vi "LABVIEW.vi"() -> ()   [LabVIEW 2017]
uses:
  <vilib>/picture/picture.llb/imagedata.ctl
  <vilib>/Instr/_visa.llb/VISA Configure Serial Port (Instr).vi
  <vilib>/Utility/file.llb/Write To Spreadsheet File (DBL).vi
panel:
  out "image data 2":T1
  out "image data":T1
  in  "Tab Control":enum32{"CONFIGURAÇÃO", "ANÁLISE", "DEBUG"}(tab)
  in  "ARQUIVO DE DADOS":path
  in  "PORTA COM":refnum<visa-resource-name>
  in  "BAUD RATE (9600)":u32=9600
  in  "TEMPO (ms)":u32
  out "new picture 2":picture
  in  "IMAGEM DA ABA CONFIGURAÇÃO":path
  in  "IMAGEM DA ABA DEBUG":path
  in  "GRAVAR":bool
  out "TEMPO (s)":dbl
  out "GRÁFICO \nTEMPERATURA":dbl(graph)
  out "TEMPERATURA":dbl
  in  "?":bool
  in  "POTÊNCIA \nRESISTÊNCIA":dbl(slide) scale=0.0..100.0
  out "?":string
  out "?":string
  out "new picture":picture
  # "ARQUIVO EM QUE OS DADOS DEVERÃO SER GRAVADOS"
  # "PORTA DE COMUNICAÇÃO UTILIZADA"
  # "VELOCIDADE DE COMUNICAÇÃO"
  # "TEMPO QUE DEFINE COM QUE PERIODICIDADE OS DADOS SÃO COLETADOS"
  # "POTÊNCIA\nRESISTÊNCIA"
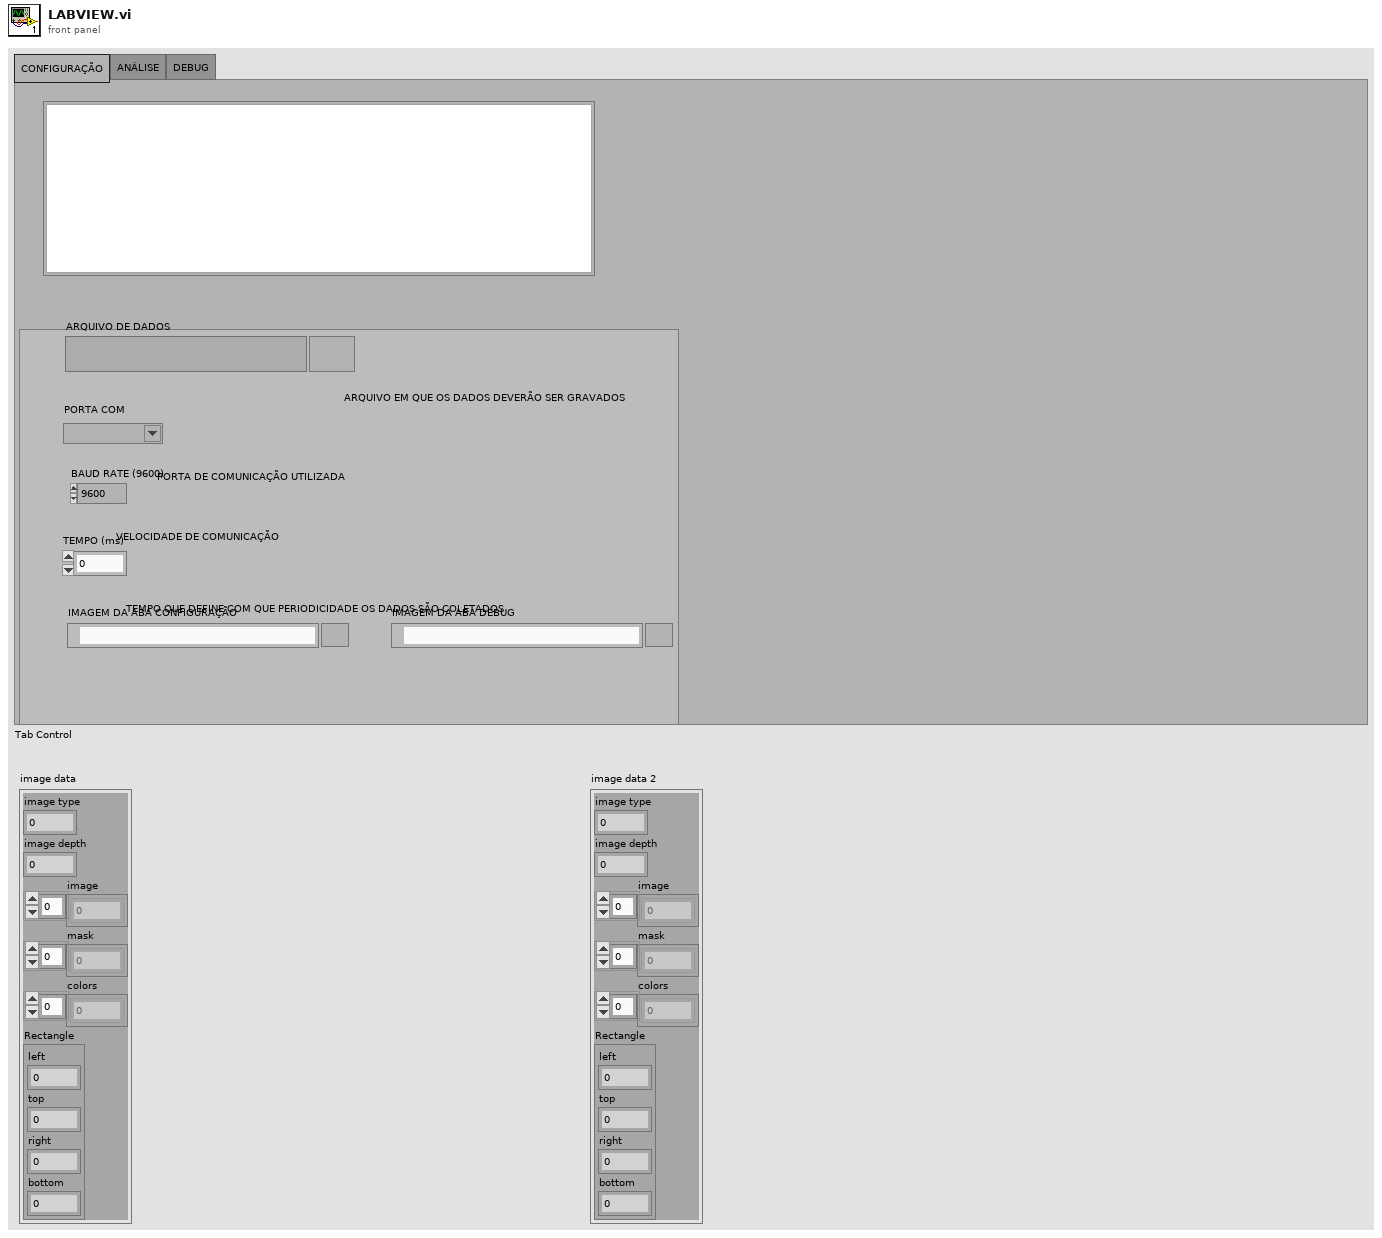
[diagram p1: front panel]
types:
  T1 = typedef "imagedata.ctl" = cluster{"image type":i32, "image depth":i32, "image":u8[], "mask":u8[], "colors":u32[], "Rectangle":cluster{"left":i16, "top":i16, "right":i16, "bottom":i16}}
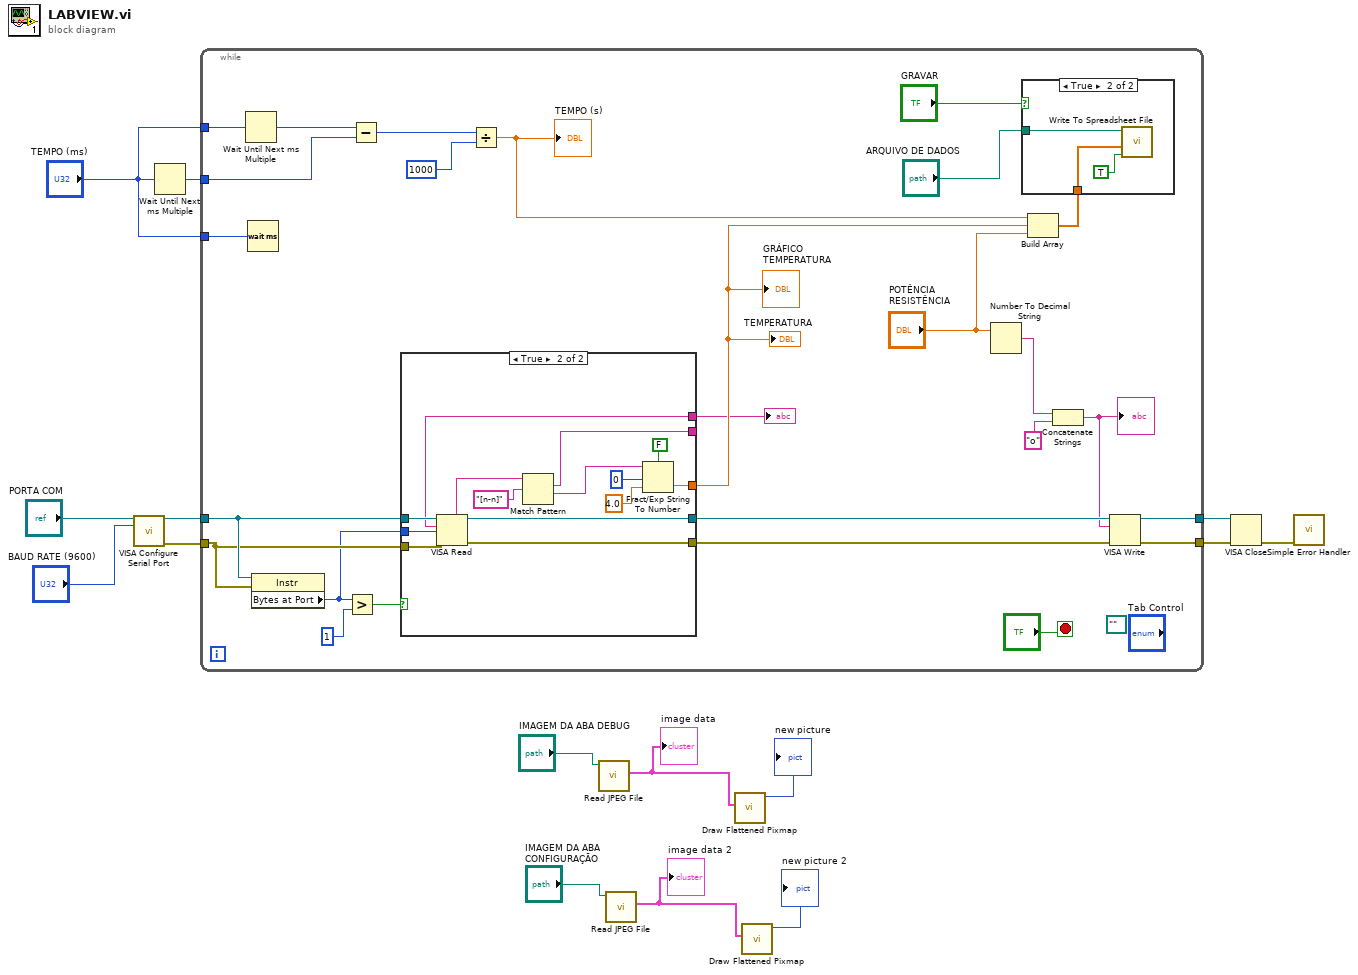
[diagram p0: block diagram]
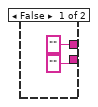
[diagram p3: hidden frame]
diagram:
  n1 = call-poly "VISA Configure Serial Port"("VISA resource name"="PORTA COM", "baud rate (9600)"="BAUD RATE (9600)") -> ("VISA resource name out"=w15:refnum<visa-resource-name>, "error out"=w14:errorcluster)  [unwired: 12 in]
  n2 = Wait Until Next ms Multiple(millisecond multiple="TEMPO (ms)") -> (millisecond timer value=w9:u32)
  n3 = while {
    tunnel: w15 -> [w39]
    tunnel: w14 -> [w38]
    tunnel: [w34] -> w11
    tunnel: [w33] -> w10
    tunnel: w9 -> [w25]
    tunnel: "TEMPO (ms)" -> [w20]
    tunnel: "TEMPO (ms)" -> [w19]
    stop <- "?" stop-if-true
    (unwired) path ""
    n4 = Wait Until Next ms Multiple(millisecond multiple=w20) -> (millisecond timer value=w28:u32)
    n5 = Wait (ms)(milliseconds to wait=w19) -> ()  [unwired: 1 out]
    n6 = property class="Instr"(reference=w39, error in=w38) -> ("Bytes at Port"=w36:u32)  [unwired: 2 out]
    n7 = Greater?(x=w36, y=u32 1) -> (0:w37:bool)
    n8 = Subtract(x=w28, y=w25) -> (x-y=w27:u32)
    n9 = case shown="True" w37 {
      tunnel: w39 -> [_ w59]
      tunnel: w38 -> [_ w58]
      tunnel: w36 -> [_ w57]
      tunnel: [_ w56] -> w35
      tunnel: [_ w55] -> w32
      tunnel: [_ w51] -> w18
      tunnel: ["" ("read buffer") w48] -> _
      tunnel: ["" ("read buffer") w47] -> w16
      frame False {
      }
      frame True {
        n10 = VISA Read(VISA resource name=w59, byte count=w57, error in (no error)=w58) -> (VISA resource name out=w56:refnum<visa-resource-name>, read buffer=w47:string, error out=w55:errorcluster)  [unwired: 1 out]
        n11 = Match Pattern(string=w47, regular expression="[n-n]") -> (match substring=w48:string, after substring=w49:string)  [unwired: 1 in, 2 out]
        n12 = Fract/Exp String To Number(use system decimal point (T)=FALSE, string=w49, offset=0, default (0 dbl)=4.0 ("default (0 DBL)")) -> (number=w51:dbl)  [unwired: 1 out]
      }
    }
    "TEMPERATURA" <- w18
    "GRÁFICO \nTEMPERATURA" <- w18
    "?" <- w16
    n13 = Divide(x=w27, y=u32 1000) -> (x/y=w22:dbl)
    "TEMPO (s)" <- w22
    n14 = Number To Decimal String(number="POTÊNCIA \nRESISTÊNCIA") -> (decimal integer string=w29:string)  [unwired: 1 in]
    n15 = Build Array(w22, w18, "POTÊNCIA \nRESISTÊNCIA") -> (w24:dbl[])
    n16 = case shown="True" "GRAVAR" {
      tunnel: "ARQUIVO DE DADOS" -> [_ w42]
      tunnel: w24 -> [_ w44]
      frame False {
      }
      frame True {
        n17 = call-poly <vilib>:"Write To Spreadsheet File.vi"("append to file? (new file:F)"=TRUE, "1D data"=w44, "file path (dialog if empty)"=w42) -> ()  [unwired: 5 in, 1 out]
      }
    }
    n18 = Concatenate Strings(w29, "o" ("string")) -> (w30:string)
    "?" <- w30
    n19 = VISA Write(VISA resource name=w35, write buffer=w30, error in (no error)=w32) -> (VISA resource name out=w34:refnum<visa-resource-name>, error out=w33:errorcluster)  [unwired: 1 out]
  }
  n20 = call <vilib>:"Read JPEG File.vi"("path to JPEG file"="IMAGEM DA ABA DEBUG") -> ("image data"=w2:T1)  [unwired: 8 in, 2 out]
  "image data" <- w2
  n21 = call <vilib>:"Read JPEG File.vi"("path to JPEG file"="IMAGEM DA ABA CONFIGURAÇÃO") -> ("image data"=w5:T1)  [unwired: 8 in, 2 out]
  "image data 2" <- w5
  n22 = call <vilib>:"Draw Flattened Pixmap.vi"("image data"=w2) -> ("new picture"=→"new picture":picture)  [unwired: 8 in]
  n23 = call <vilib>:"Draw Flattened Pixmap.vi"("image data"=w5) -> ("new picture"=→"new picture 2":picture)  [unwired: 8 in]
  n24 = VISA Close(VISA resource name=w11, error in (no error)=w10) -> (error out=w12:errorcluster)
  n25 = call <vilib>:"Simple Error Handler.vi"("error in (no error)"=w12) -> ()  [unwired: 4 in, 5 out]
